vi "XML.Configuration.Generate.vi"(8 "error in":errorcluster, 9 "Root name":string="HWConfigFile", 10 "Config":T1[](array[typedef]), 11 "XML file path":path=path "C:/Projects/TM-OS/trunk/Design/XML_HW_config2.xml") -> (0 "error out":errorcluster)   [LabVIEW 2019, in "Tools.lvlib"]
uses:
  Tools.lvlib
  LibXML/LibXML.lvlib
  Modules/Sequences_Management/SubVIs/ConfigurationWizard/controls/ConfigurationWIzard.Config.ctl
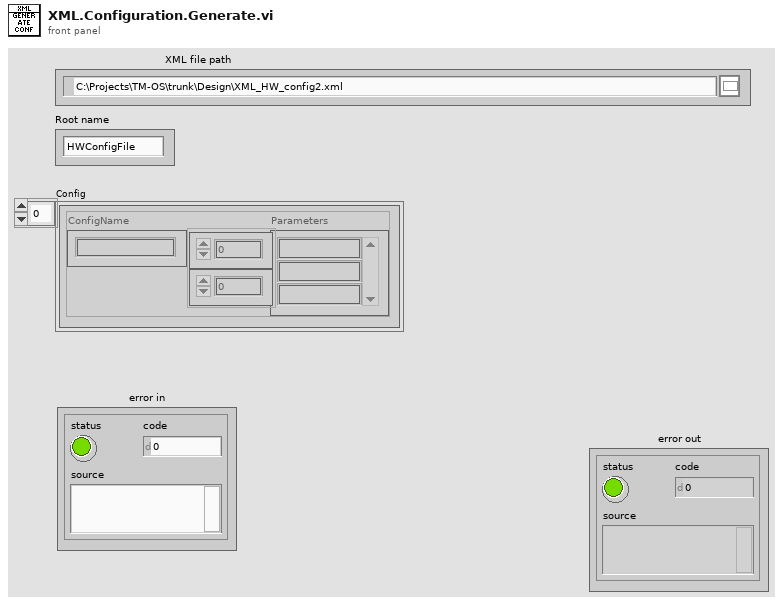
[diagram p1: front panel]
types:
  T1 = typedef "ConfigurationWIzard.Config.ctl" = cluster{"ConfigName":string, "Parameters":string[][]}
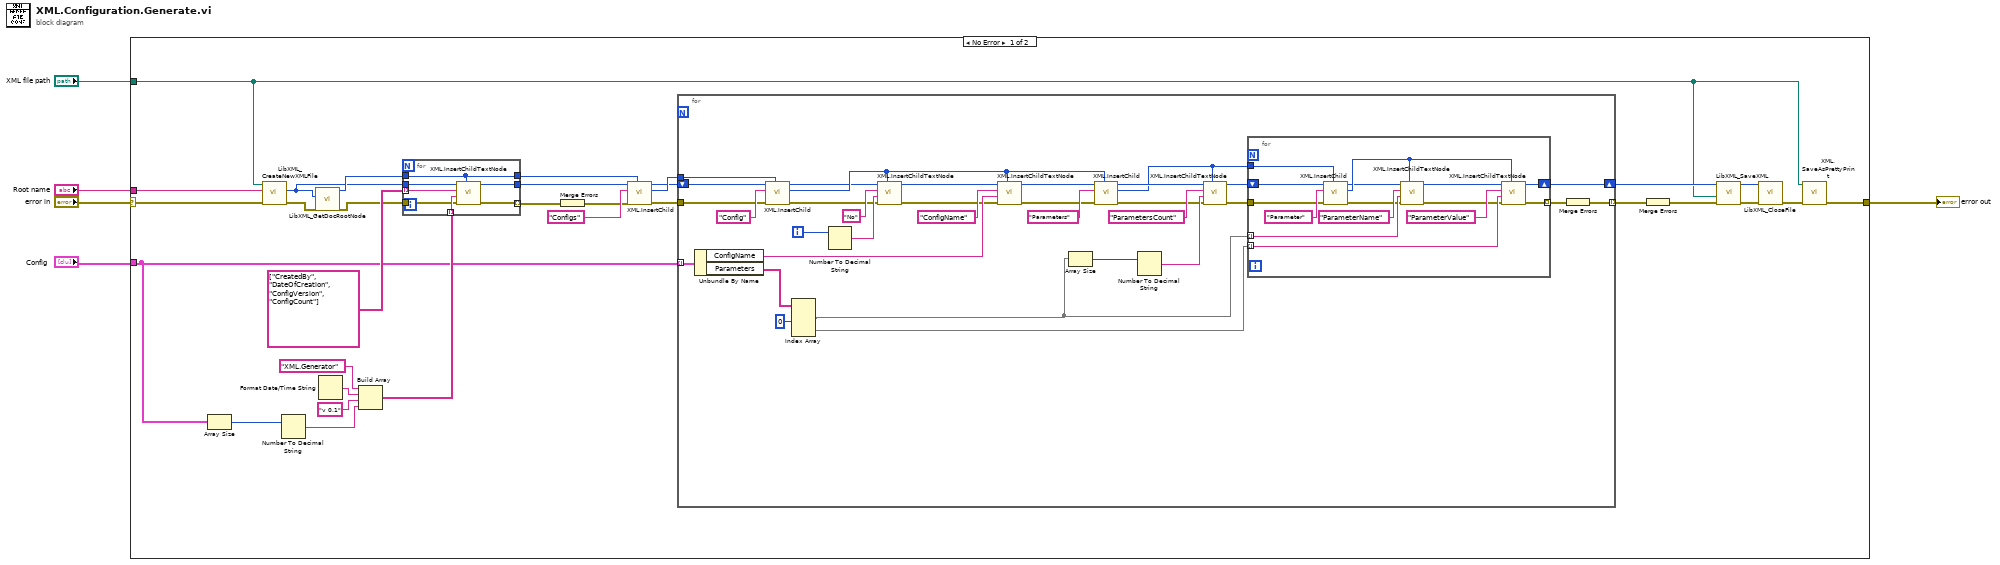
[diagram p0: block diagram]
diagram:
  n1 = case shown="No Error" "error in" {
    selector: "error in" -> [w18 w91]
    tunnel: "Config" -> [w23 _]
    tunnel: [w12 w91] -> w3
    tunnel: "Root name" -> [w13 _]
    tunnel: "XML file path" -> [w6 _]
    frame No Error {
      n2 = Array Size(array=w23) -> (size(s)=w30:i32)
      n3 = call "LibXML_CreateNewXMLFile.vi"("error in"=w18, "Root element name"=w13, "file path"=w6) -> ("error out"=w17:errorcluster, "new doc out"=w15:u32)  [unwired: 6 in, 1 out]
      n4 = Number To Decimal String(number=w30) -> (decimal integer string=w29:string)  [unwired: 1 in]
      n5 = call "LibXML_GetDocRootNode.vi"("error in"=w17, "doc"=w15) -> ("error out"=w14:errorcluster, "root node out"=w16:u32)  [unwired: 8 in]
      n6 = Format Date/Time String() -> (date/time string=w32:string)  [unwired: 3 in]
      n7 = Build Array("XML.Generator" ("Tag Name"), w32, "v 0.1" ("element"), w29) -> (w33:string[])
      n8 = for {
        tunnel: string[] ["CreatedBy", "DateOfCreation", "ConfigVersion", "ConfigCount"] -> [w42] mode=indexing
        tunnel: w15 -> [w39]
        tunnel: w16 -> [w38]
        tunnel: w33 -> [w41] mode=indexing
        tunnel: [w40] -> w26
        tunnel: [w38] -> w24
        tunnel: w14 -> [w37]
        tunnel: [w36] -> w22 mode=indexing
        n9 = call "XML.InsertChildTextNode.vi"("parent"=w38, "error in"=w37, "text"=w41, "name"=w42, "doc"=w39) -> ("error out"=w36:errorcluster, "doc out"=w40:u32)  [unwired: 5 in]
      }
      n10 = Merge Errors(w22) -> (w21:errorcluster)
      n11 = call "XML.InsertChild.vi"("parent"=w24, "error in"=w21, "name"="Configs" ("Tag Name"), "doc"=w26) -> ("error out"=w20:errorcluster, "new node"=w28:u32, "doc out"=w25:u32)  [unwired: 5 in]
      n12 = for {
        tunnel: w23 -> [w55] mode=indexing
        tunnel: w28 -> [w74]
        shift-right: [w72] -> w7
        shift-left: w25 -> [w73]
        tunnel: w20 -> [w50]
        tunnel: [w43] -> w19 mode=indexing
        i -> [w75]
        n13 = Unbundle By Name(w55) -> ("ConfigName"=w56:string, "Parameters"=w54:string[][])
        n14 = call "XML.InsertChild.vi"("parent"=w74, "error in"=w50, "name"="Config" ("Tag Name"), "doc"=w73) -> ("error out"=w49:errorcluster, "new node"=w63:u32, "doc out"=w60:u32)  [unwired: 5 in]
        n15 = Index Array(array=w54, index (col) #1=0 ("disabled index (col)")) -> (element #1=w53:string[], element #2=w52:string[])  [unwired: 3 in]
        n16 = Number To Decimal String(number=w75) -> (decimal integer string=w70:string)  [unwired: 1 in]
        n17 = call "XML.InsertChildTextNode.vi"("parent"=w63, "error in"=w49, "text"=w70, "name"="No" ("Tag Name"), "doc"=w60) -> ("error out"=w48:errorcluster, "doc out"=w59:u32)  [unwired: 5 in]
        n18 = call "XML.InsertChildTextNode.vi"("parent"=w63, "error in"=w48, "text"=w56, "name"="ConfigName", "doc"=w59) -> ("error out"=w47:errorcluster, "doc out"=w61:u32)  [unwired: 5 in]
        n19 = Array Size(array=w53) -> (size(s)=w67:i32)
        n20 = call "XML.InsertChild.vi"("parent"=w63, "error in"=w47, "name"="Parameters" ("Tag Name"), "doc"=w61) -> ("error out"=w46:errorcluster, "new node"=w57:u32, "doc out"=w62:u32)  [unwired: 5 in]
        n21 = Number To Decimal String(number=w67) -> (decimal integer string=w66:string)  [unwired: 1 in]
        n22 = call "XML.InsertChildTextNode.vi"("parent"=w57, "error in"=w46, "text"=w66, "name"="ParametersCount", "doc"=w62) -> ("error out"=w45:errorcluster, "doc out"=w58:u32)  [unwired: 5 in]
        n23 = for {
          tunnel: w57 -> [w87]
          shift-right: [w82] -> w72
          shift-left: w58 -> [w86]
          tunnel: w53 -> [w81] mode=indexing
          tunnel: w52 -> [w80] mode=indexing
          tunnel: w45 -> [w79]
          tunnel: [w76] -> w44 mode=indexing
          n24 = call "XML.InsertChild.vi"("parent"=w87, "error in"=w79, "name"="Parameter" ("Tag Name"), "doc"=w86) -> ("error out"=w78:errorcluster, "new node"=w85:u32, "doc out"=w84:u32)  [unwired: 5 in]
          n25 = call "XML.InsertChildTextNode.vi"("parent"=w85, "error in"=w78, "text"=w81, "name"="ParameterName", "doc"=w84) -> ("error out"=w77:errorcluster, "doc out"=w83:u32)  [unwired: 5 in]
          n26 = call "XML.InsertChildTextNode.vi"("parent"=w85, "error in"=w77, "text"=w80, "name"="ParameterValue", "doc"=w83) -> ("error out"=w76:errorcluster, "doc out"=w82:u32)  [unwired: 5 in]
        }
        n27 = Merge Errors(w44) -> (w43:errorcluster)
      }
      n28 = Merge Errors(w19) -> (w11:errorcluster)
      n29 = call "LibXML_SaveXML.vi"("error in"=w11, "file path (dialog if empty)"=w6, "doc"=w7) -> ("error out"=w10:errorcluster, "doc copy out"=w8:u32)  [unwired: 6 in, 1 out]
      n30 = call "LibXML_CloseFile.vi"("error in"=w10, "doc"=w8) -> ("error out"=w9:errorcluster)  [unwired: 9 in]
      n31 = call "XML.SaveAsPrettyPrint.vi"("error in (no error)"=w9, "XML file path"=w6) -> ("error out"=w12:errorcluster)  [unwired: 9 in]
    }
    frame Error {
    }
  }
  "error out" <- w3
